vi "Close.vi"(8 "error in (no error)":errorcluster, 11 "VISA resource name":refnum<visa-resource-name>) -> (0 "error out":errorcluster)   [LabVIEW 2017, in "Drivers.lvlib" / "ASI TG-1000.lvlib"]
doc: "Performs an instrument error query before terminating the software connection to the instrument."
uses:
  ASI TG-1000.lvlib
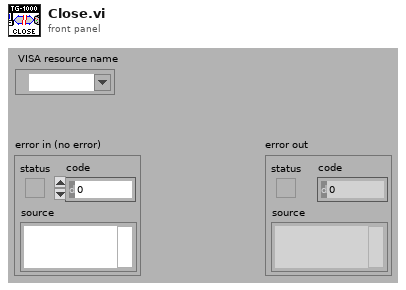
[diagram p1: front panel]
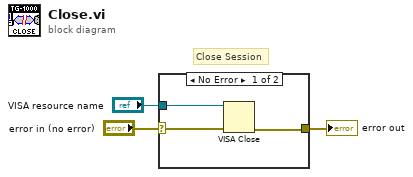
[diagram p0: block diagram]
diagram:
  # "Close Session"
  n1 = case shown="No Error" "error in (no error)" {
    selector: "error in (no error)" -> [w4 w7]
    tunnel: "VISA resource name" -> [w6 _]
    tunnel: [w5 w7] -> w2
    frame No Error {
      n2 = VISA Close(VISA resource name=w6, error in (no error)=w4) -> (error out=w5:errorcluster)
    }
    frame Error {
    }
  }
  "error out" <- w2
